vi "Command Find Tote.vi"(2 "Input Robot System Funtions":T1, 3 "Cmd Parameter 1":dbl, 4 "Cmd Parameter 2":dbl, 5 "Startup":bool) -> (0 "Output Robot System Functions":T1, 1 "Completed":bool)   [LabVIEW 2014]
uses:
  Subsystems VIs/Robot Commands.ctl
  Command Execution State.ctl
  Global Variables/Sensor Data (Edited).vi
  Global Variables/Settings.vi
panel:
  out "Driver Switch 2":bool
  out "PID Tracking":cluster{"Goal Wheel Position":dbl, dbl}(graph)={"Goal Wheel Position"=0.0, -90.17571233858979}
  # "Sample robot\ncontrol output.\nReplace with \nactual teleop \ncontrol signal \nstructure."
  # "Field Centric"
  # "Field Centric"
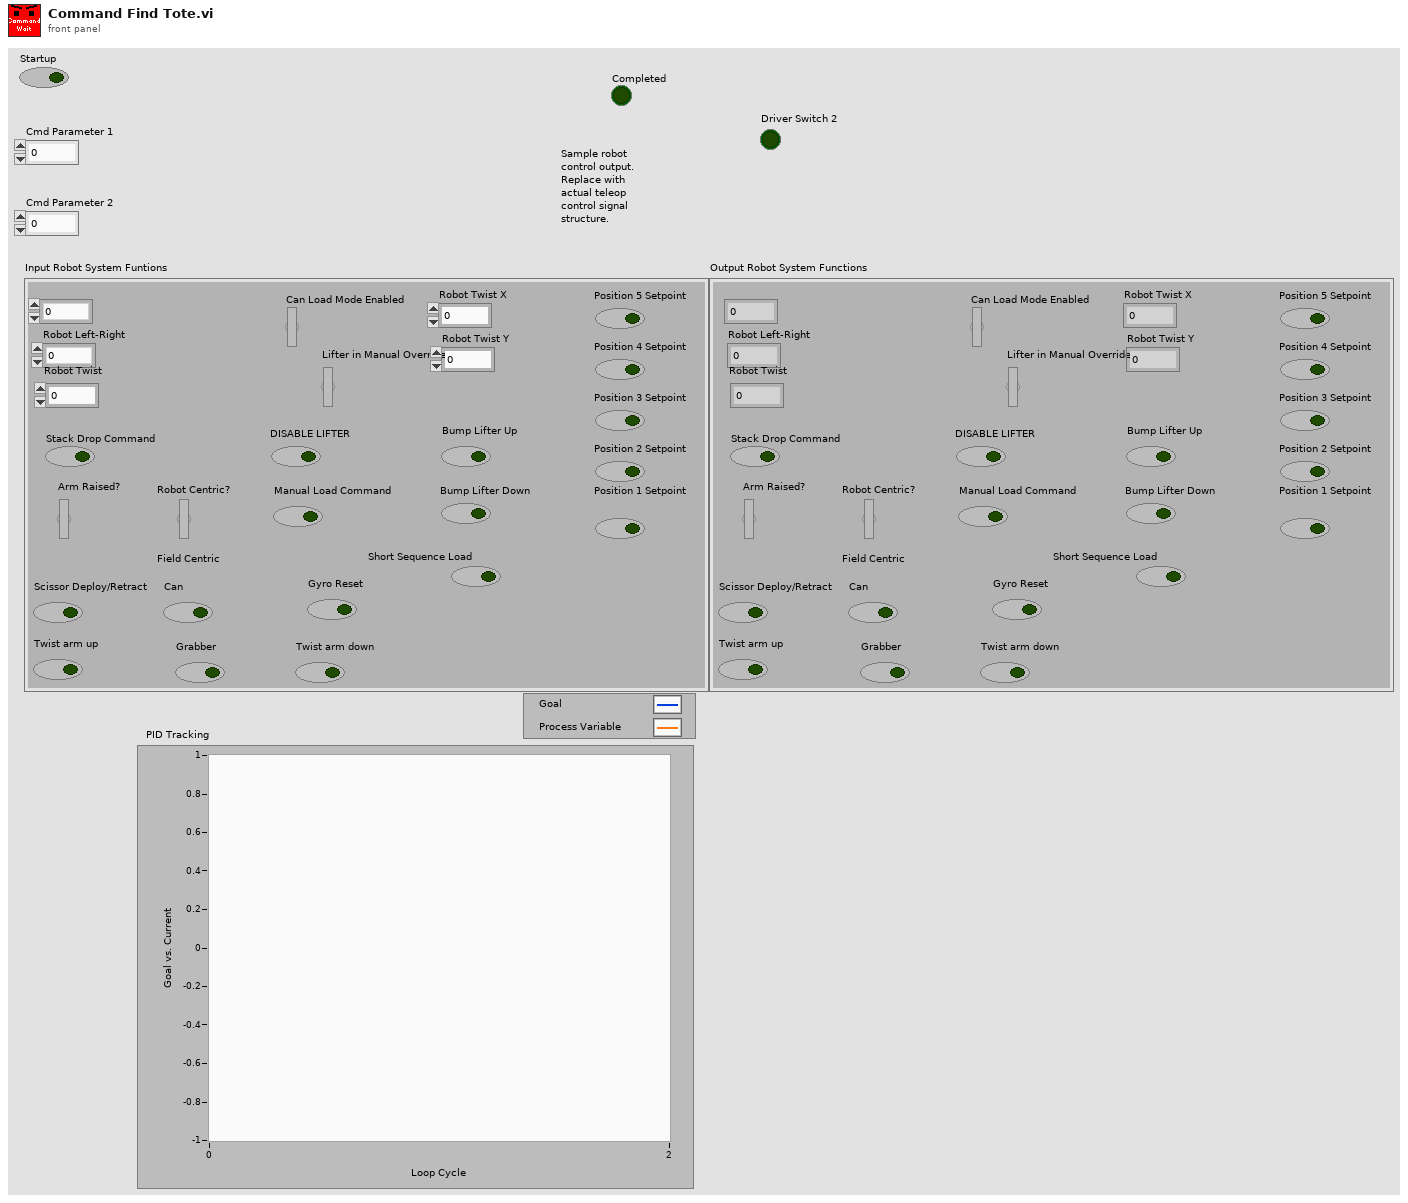
[diagram p1: front panel]
types:
  T1 = typedef "Robot Commands.ctl" = cluster{"Robot Forward-Reverse":dbl, "Robot Left-Right":dbl, "Robot Twist":dbl, "Can Load Mode Enabled":bool, "Lifter in Manual Override?":bool, "Stack Drop Command":bool, "Arm Raised?":bool, "DISABLE LIFTER":bool, "Position 1 Setpoint":bool, "Position 2 Setpoint":bool, "Position 3 Setpoint":bool, "Position 4 Setpoint":bool, "Position 5 Setpoint":bool, "Bump Lifter Down":bool, "Bump Lifter Up":bool, "Manual Load Command":bool, "Robot Centric?":bool, "Scissor Deploy/Retract":bool, "Grabber":bool, "Can":bool, "Twist arm up":bool, "Gyro Reset":bool, "Twist arm down":bool, "Short Sequence Load":bool, "Robot Twist X":dbl, "Robot Twist Y":dbl}
  T2 = typedef "Command Execution State.ctl" = enum16{"Initialize", "Execute", "Finish"}
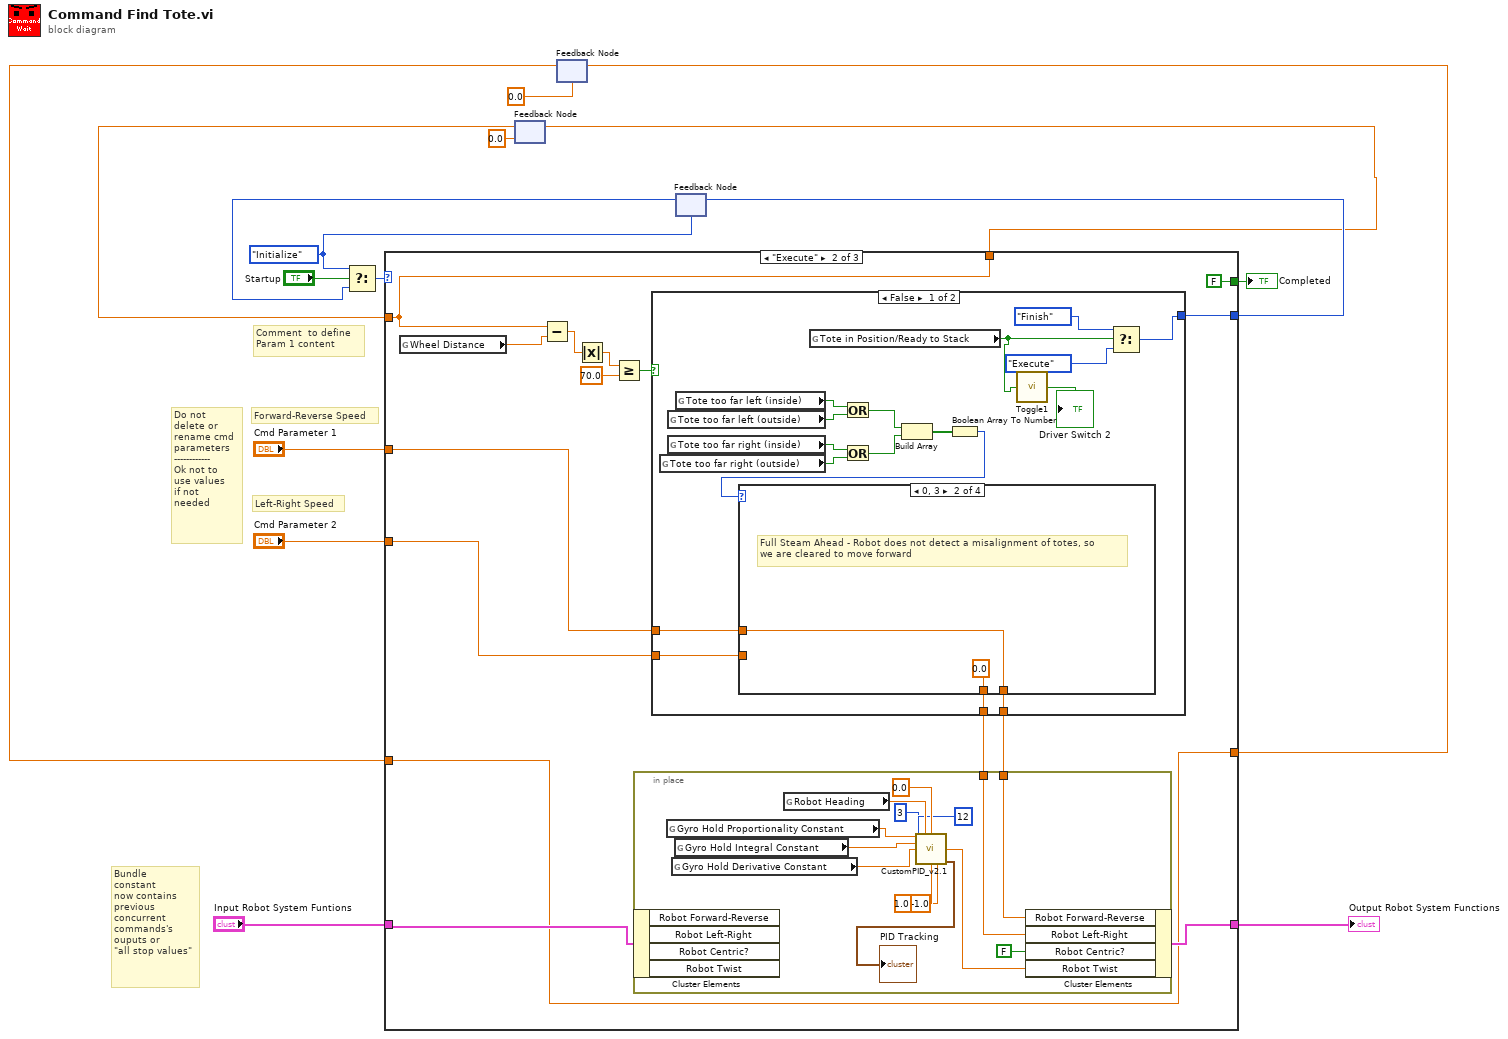
[diagram p0: block diagram]
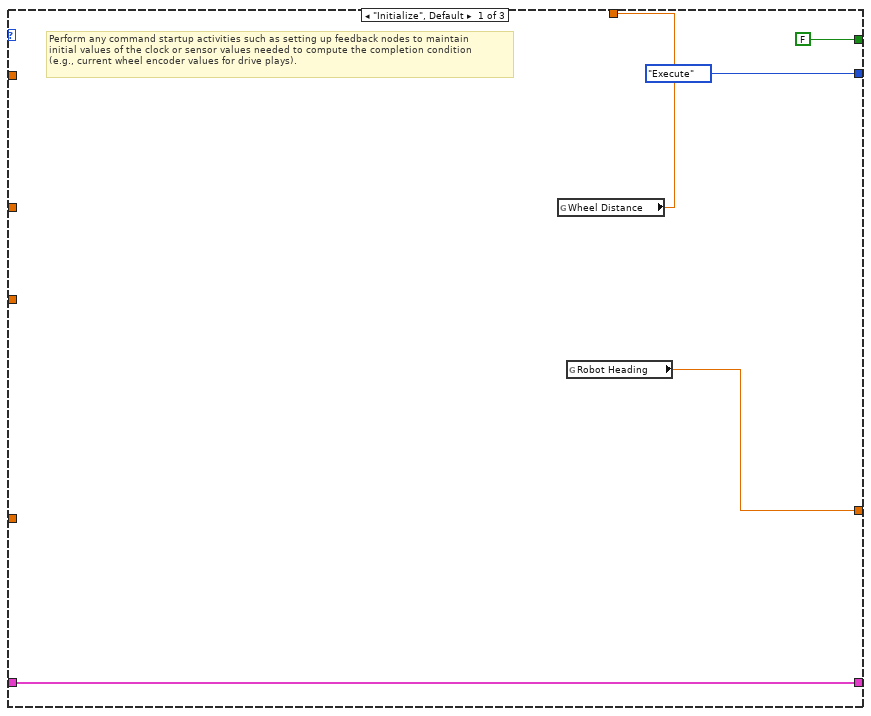
[diagram p2: hidden frame]
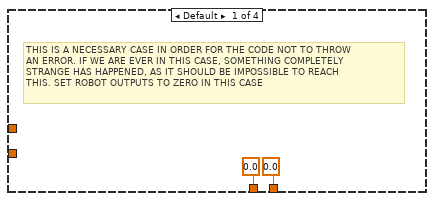
[diagram p3: hidden frame]
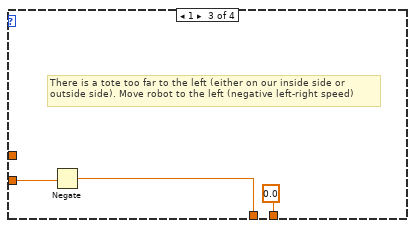
[diagram p4: hidden frame]
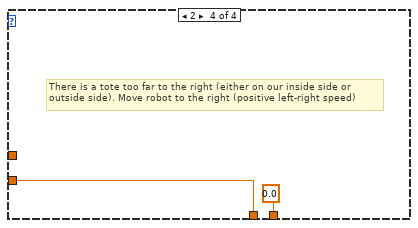
[diagram p5: hidden frame]
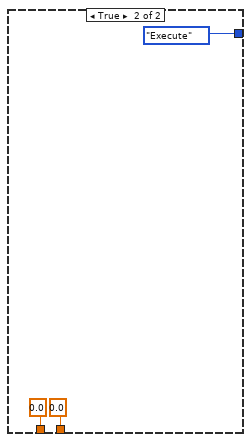
[diagram p6: hidden frame]
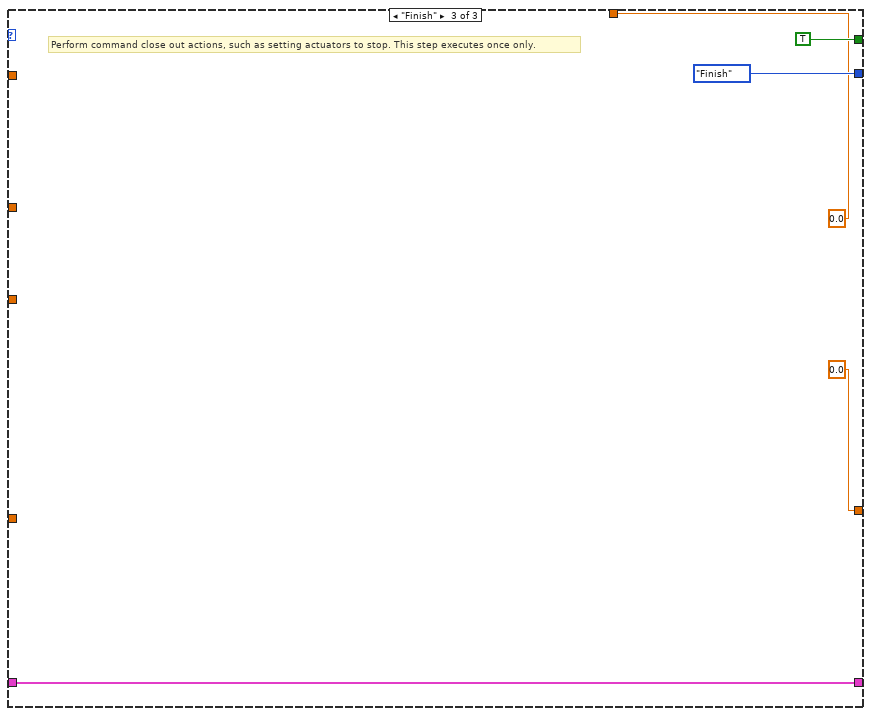
[diagram p7: hidden frame]
diagram:
  w11 = Command_Execution_State."Initialize" ("Play State")
  # "Forward-Reverse Speed"
  # "Bundle \nconstant\nnow contains\nprevious \nconcurrent\ncommands's\nouputs or\n\"all stop values\""
  # "Do not \ndelete or\nrename cmd\nparameters\n------------\nOk not to \nuse values\nif not \nneeded"
  # "Left-Right Speed"
  # "Comment  to define\nParam 1 content"
  n1 = feedback #1(0.0 ("Wheel Distance")) -> (w6:dbl)
  n2 = feedback #2(0.0 ("Wheel Distance")) -> (w3:dbl)
  n3 = feedback #3(w11) -> (w12:T2)
  n4 = Select(t=w11, s="Startup", f=w12) -> (s? t:f=w16:T2)
  n5 = case shown="\"Execute\"" w16 {
    tunnel: [FALSE FALSE TRUE] -> w14
    tunnel: [Command_Execution_State."Execute" ("Play State") w22 Command_Execution_State."Finish" ("f")] -> w13
    tunnel: "Cmd Parameter 1" -> [_ w26 _]
    tunnel: "Cmd Parameter 2" -> [_ w25 _]
    tunnel: [w19 w35 w80] -> w7
    tunnel: "Input Robot System Funtions" -> [w19 w36 w80]
    tunnel: [w18 w30 0.0 ("Wheel Distance")] -> w1
    tunnel: w6 -> [_ w30 _]
    tunnel: [w17 w28 0.0 ("Wheel Distance")] -> w4
    tunnel: w3 -> [_ w28 _]
    frame "Initialize", Default {
      # "Perform any command startup activities such as setting up feedback nodes to maintain \ninitial values of the clock or sensor values needed to compute the completion condition\n(e.g., current wheel encoder values for drive plays)."
      n6 = global read "Sensor Data (Edited).vi" "Wheel Distance"() -> (w18:dbl)
      n7 = global read "Sensor Data (Edited).vi" "Robot Heading"() -> (w17:dbl)
    }
    frame "Execute" {
      n8 = global read "Sensor Data (Edited).vi" "Wheel Distance"() -> (w34:dbl)
      n9 = Subtract(x=w30, y=w34) -> (x-y=w33:dbl)
      n10 = Absolute Value(x=w33) -> (abs(x)=w32:dbl)
      n11 = Greater Or Equal?(x=w32, y=70.0) -> (x >= y?=w27:bool)
      n12 = case shown="False" w27 {
        tunnel: w26 -> [w45 _]
        tunnel: w25 -> [w44 _]
        tunnel: [w43 0.0 ("Cmd Parameter 1")] -> w24
        tunnel: [w42 0.0 ("Cmd Parameter 2")] -> w23
        tunnel: [w39 Command_Execution_State."Execute" ("f")] -> w22
        frame False {
          n13 = global read "Sensor Data (Edited).vi" "Tote too far right (outside)"() -> (w52:bool)
          n14 = global read "Sensor Data (Edited).vi" "Tote too far left (outside)"() -> (w51:bool)
          n15 = global read "Sensor Data (Edited).vi" "Tote too far right (inside)"() -> (w53:bool)
          n16 = global read "Sensor Data (Edited).vi" "Tote too far left (inside)"() -> (w50:bool)
          n17 = global read "Sensor Data (Edited).vi" "Tote in Position/Ready to Stack"() -> (w38:bool)
          n18 = Or(x=w50, y=w51) -> (x .or. y?=w49:bool)
          n19 = Or(x=w53, y=w52) -> (x .or. y?=w48:bool)
          n20 = Build Array(w49, w48) -> (w47:bool[])
          n21 = Boolean Array To Number(Boolean array=w47) -> (number=w46:u32)
          n22 = case shown="0, 3" w46 {
            tunnel: w45 -> [_ w57 _ _]
            tunnel: w44 -> [_ _ w60 w62]
            tunnel: [0.0 ("Cmd Parameter 1") w57 0.0 ("Cmd Parameter 1") 0.0 ("Cmd Parameter 1")] -> w43
            tunnel: [0.0 ("Cmd Parameter 2") 0.0 ("Cmd Parameter 2") w59 w62] -> w42
            frame Default {
              # "THIS IS A NECESSARY CASE IN ORDER FOR THE CODE NOT TO THROW\nAN ERROR. IF WE ARE EVER IN THIS CASE, SOMETHING COMPLETELY \nSTRANGE HAS HAPPENED, AS IT SHOULD BE IMPOSSIBLE TO REACH \nTHIS. SET ROBOT OUTPUTS TO ZERO IN THIS CASE"
            }
            frame 0, 3 {
              # "Full Steam Ahead - Robot does not detect a misalignment of totes, so\nwe are cleared to move forward"
            }
            frame 1 {
              # "There is a tote too far to the left (either on our inside side or\noutside side). Move robot to the left (negative left-right speed)"
              n23 = Negate(x=w60) -> (-x=w59:dbl)
            }
            frame 2 {
              # "There is a tote too far to the right (either on our inside side or\noutside side). Move robot to the right (positive left-right speed)"
            }
          }
          n24 = call "Toggle1.vi"("Boolean"=w38) -> ("Driver Switch 2"=→"Driver Switch 2":bool)
          n25 = Select(t=Command_Execution_State."Finish" ("f"), s=w38, f=Command_Execution_State."Execute") -> (s? t:f=w39:T2)
        }
        frame True {
        }
      }
      n26 = in-place {
        in-place-border: w24 -> [w67]
        in-place-border: w23 -> [w66]
        n27 = in-place-cluster #4(w36) -> ()  [unwired: 4 out]
        n28 = global read "Settings.vi" "Gyro Hold Proportionality Constant"() -> (w71:dbl)
        n29 = global read "Settings.vi" "Gyro Hold Derivative Constant"() -> (w69:dbl)
        n30 = global read "Settings.vi" "Gyro Hold Integral Constant"() -> (w70:dbl)
        n31 = global read "Sensor Data (Edited).vi" "Robot Heading"() -> (w77:dbl)
        n32 = call "CustomPID_v2.1.vi"("Kp"=w71, "Process Variable"=w77, "Goal"=0.0 ("Setpoint"), "Ki"=w70, "Kd"=w69, "N-Diff"=3, "N-Int"=12, "Max Ouput"=1.0, "Min Output"=-1.0) -> ("Command"=w78:dbl, "PID Tracking"=→"PID Tracking":cluster{"Goal Wheel Position":dbl, dbl})  [unwired: 4 in, 1 out]
        n33 = in-place-cluster #4("Robot Forward-Reverse"=w67, "Robot Left-Right"=w66, "Robot Centric?"=FALSE, "Robot Twist"=w78) -> (w35:T1)
      }
    }
    frame "Finish" {
      # "Perform command close out actions, such as setting actuators to stop. This step executes once only."
    }
  }
  "Completed" <- w14
  "Output Robot System Functions" <- w7
  n34 = feedback-in #1(w1) -> ()
  n35 = feedback-in #2(w4) -> ()
  n36 = feedback-in #3(w13) -> ()
